vi "stim_LED_and_save_stim_instances_older_LabView2014_SK.vi"() -> ()   [LabVIEW 2014]
uses:
  <vilib>/Utility/file.llb/Write To Spreadsheet File (string).vi
panel:
  in  "Time bin dur. (ms)":u32
  in  "number of stims":dbl
  in  "Power ON":dbl
  in  "Time ON (sec)":dbl
  in  "Power OFF":dbl
  in  "Time OFF (sec)":dbl
  out "Error":string
  in  "OK Button":bool
  out "stim timestamp":timestamp
  out "Waveform Chart":dbl(graph)
  # "Press OK button once to deliver stims with defined number of stims"
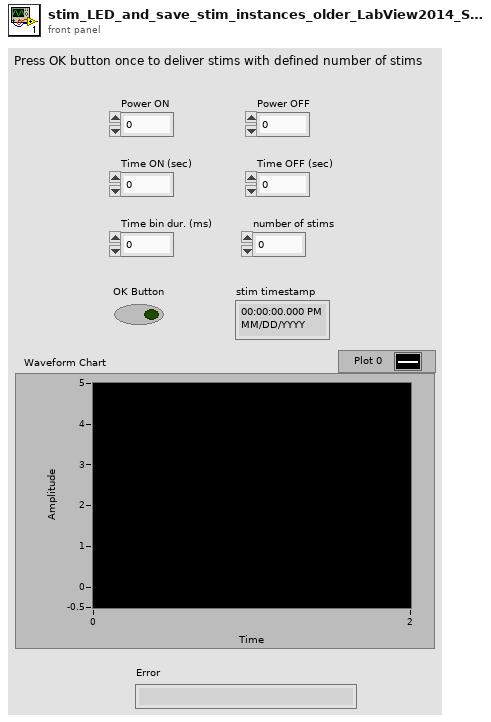
[diagram p1: front panel]
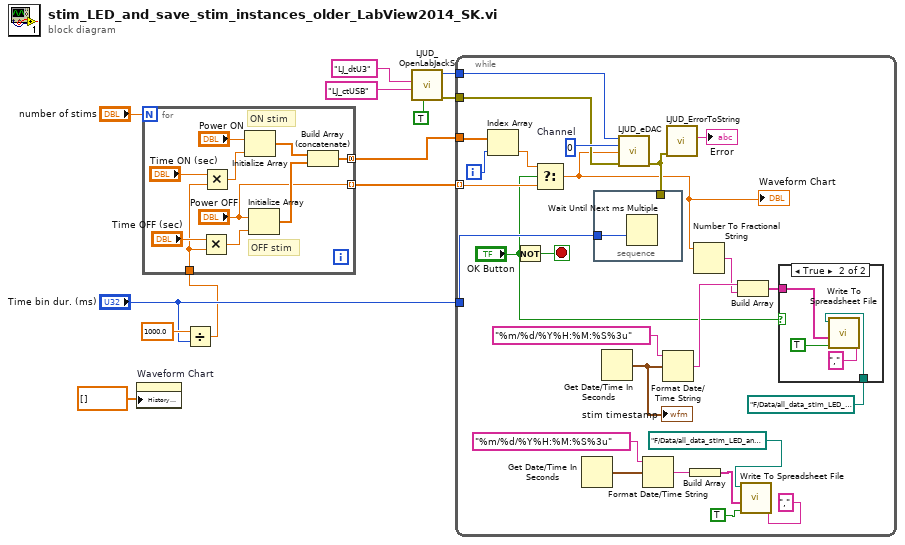
[diagram p0: block diagram]
diagram:
  n1 = property on="Waveform Chart" class="WFChart (strict)"("History Data"=dbl[] []) -> ()  [unwired: 2 in, 2 out]
  n2 = Divide(x=1000.0, y="Time bin dur. (ms)") -> (x/y=w3:dbl)
  n3 = for {
    N: "number of stims" -> [_]
    tunnel: [w19] -> w1 mode=concatenating
    tunnel: ["Power OFF"] -> w6 mode=indexing
    tunnel: w3 -> [w14]
    # "ON stim"
    # "OFF stim"
    n4 = Multiply(x="Time OFF (sec)", y=w14) -> (x*y=w13:dbl)
    n5 = Multiply(x="Time ON (sec)", y=w14) -> (x*y=w17:dbl)
    n6 = Initialize Array("Power ON", w17) -> (w21:dbl[])
    n7 = Initialize Array("Power OFF", w13) -> (w22:dbl[])
    n8 = Build Array (concatenate)(w21, w22) -> (w19:dbl[])
  }
  n9 = call "LJUD_OpenLabJackS.vi"("FirstFound"=TRUE, "ConnectionType"="LJ_ctUSB", "DeviceType"="LJ_dtU3") -> ("error out"=w9:errorcluster, "Handle"=w8:i32)  [unwired: 6 in, 1 out]
  n10 = while {
    tunnel: w1 -> [w42]
    tunnel: w9 -> [w43]
    tunnel: w8 -> [w45]
    tunnel: w6 -> [w39] mode=indexing
    tunnel: "Time bin dur. (ms)" -> [w33]
    i -> [w44]
    stop <- w41 stop-if-true
    w47 = 0  # Channel
    n11 = Index Array(array=w42, index=w44) -> (element=w40:dbl)
    n12 = Not(x="OK Button") -> (.not. x?=w41:bool)
    n13 = Select(t=w40, s="OK Button", f=w39) -> (s? t:f=w32:dbl)
    "Waveform Chart" <- w32
    n14 = Get Date/Time In Seconds() -> (seconds since 1Jan1904=w30:timestamp)
    n15 = Get Date/Time In Seconds() -> (seconds since 1Jan1904=w38:timestamp)
    "stim timestamp" <- w38
    n16 = call "LJUD_eDAC.vi"("Handle In"=w45, "Channel"=w47, "Voltage"=w32, "error in"=w43) -> ("error out"=w46:errorcluster)  [unwired: 10 in, 1 out]
    n17 = stacked-sequence {
      tunnel: w33 -> [w53]
      tunnel: w46 -> [_]
      frame #0 {
        n18 = Wait Until Next ms Multiple(millisecond multiple=w53) -> ()  [unwired: 1 out]
      }
    }
    n19 = Format Date/Time String(time format string (%c)="%m/%d/%Y%H:%M:%S%3u", seconds (now)=w30) -> (date/time string=w31:string)  [unwired: 1 in]
    n20 = Format Date/Time String(time format string (%c)="%m/%d/%Y%H:%M:%S%3u", seconds (now)=w38) -> (date/time string=w35:string)  [unwired: 1 in]
    n21 = call "LJUD_ErrorToString.vi"("error in"=w46) -> ("String"=→"Error":string)  [unwired: 10 in]
    n22 = Build Array(w31) -> (w26:string[])
    n23 = Number To Fractional String(number=w32) -> (F-format string=w34:string)  [unwired: 3 in]
    n24 = Build Array(w35, w34) -> (w28:string[])
    n25 = call-poly <vilib>:"Write To Spreadsheet File.vi"("delimiter (\\t)"="," ("delimiter (\\t)"), "append to file? (new file:F)"=TRUE, "1D data"=w26, "file path (dialog if empty)"=path "F:/Data/all_data_stim_LED_and_save_stim_instances/excel_files/all_time_data.csv") -> ()  [unwired: 4 in, 1 out]
    n26 = case shown="True" "OK Button" {
      tunnel: path "F:/Data/all_data_stim_LED_and_save_stim_instances/excel_files/stim_data.csv" ("file path (dialog if empty)") -> [_ w50]
      tunnel: w28 -> [_ w51]
      frame False {
      }
      frame True {
        n27 = call-poly <vilib>:"Write To Spreadsheet File.vi"("delimiter (\\t)"="," ("delimiter (\\t)"), "append to file? (new file:F)"=TRUE, "1D data"=w51, "file path (dialog if empty)"=w50) -> ()  [unwired: 4 in, 1 out]
      }
    }
  }
